vi "VariaveisParametros.vi"() -> ()   [LabVIEW 2019]
panel:
  in  "TaxaTransmissãoDados":dbl
  in  "TempoAquisicao":dbl
  in  "TempoEntrePontos":dbl
  in  "Pontos":dbl[](array[numeric])
  in  "ListaMedicaoPorta":string[][](array[string])
  in  "GeracaoSelecionada":string
  out "SelecionarGeracao":bool
  in  "OndaSelecionada":T1(ring)
  in  "TipoGeraçãoSelect":u16(ring) items=["Modo Continuo", "Limitado por tempo", "Ponto por ponto"]
  in  "TempoTeste":dbl
  out "InfoContinuo":T2={"TempRampas"=0.0, "PicoMax"=0.0, "TextUnidMed"="segundos"}
  out "InfoInSenoide":T3
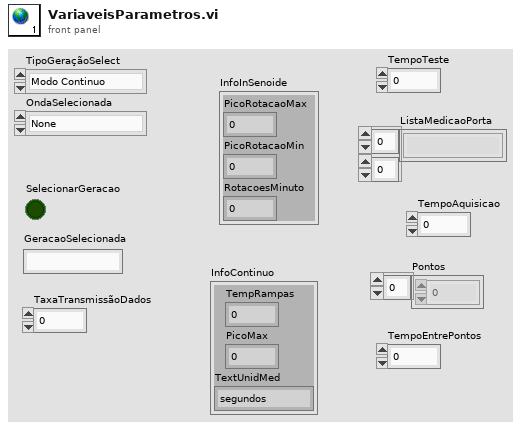
[diagram p1: front panel]
types:
  T1 = enum16{"None", "Continua", "Senoidal", "Quadrada"}
  T2 = cluster{"TempRampas":dbl, "PicoMax":dbl, "TextUnidMed":string}
  T3 = cluster{"PicoRotacaoMax":dbl, "PicoRotacaoMin":dbl, "RotacoesMinuto":dbl}
diagram:
